vi "Set Color by Argb.vi"(8 "error in (no error)":errorcluster caption="错误输入（无错误）", 9 "blue":i32, 10 "green":i32, 11 "red":i32) -> (0 "error out":errorcluster caption="错误输出", 3 "FromArgb":refnum<k24>)   [LabVIEW 2012, in "Color.lvclass"]
uses:
  Color.lvclass
  System.Drawing
panel:
  in  "alpha":i32
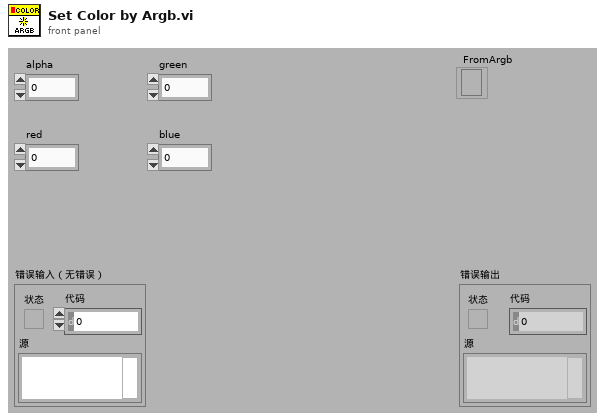
[diagram p1: front panel]
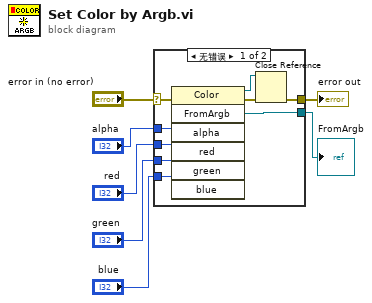
[diagram p0: block diagram]
diagram:
  n1 = case shown="无错误" "error in (no error)" {
    selector: "error in (no error)" -> [w16 w17]
    tunnel: [w15 w17] -> w6
    tunnel: "alpha" -> [w14 _]
    tunnel: "red" -> [w13 _]
    tunnel: "green" -> [w12 _]
    tunnel: "blue" -> [w11 _]
    tunnel: [w8 _] -> w1
    frame No Error {
      n2 = invoke class="Color" method="FromArgb"(error in=w16, "alpha"=w14, "red"=w13, "green"=w12, "blue"=w11) -> (reference out=w10:refnum<k24>, error out=w9:errorcluster, "FromArgb"=w8:refnum<k24>)  [unwired: 2 in, 4 out]
      n3 = Close Reference(reference=w10, error in (no error)=w9) -> (error out=w15:errorcluster)
    }
    frame Error {
    }
  }
  "error out" <- w6
  "FromArgb" <- w1
